vi "Acquire Test.vi"() -> ()   [LabVIEW 2018]
panel:
  out "Waveform Graph":waveform(dbl)(graph)
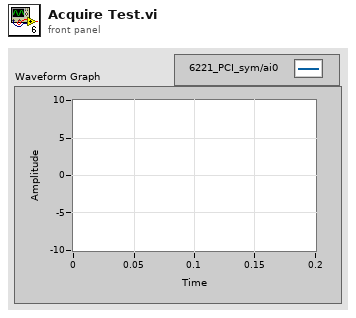
[diagram p1: front panel]
types:
  T1 = typedef "daqtypedef.ctl" = cluster{"PhysicalChanName":tag, "AI.Max":dbl, "AI.Min":dbl, "SampQuant.SampPerChan":dbl, "SampClk.Rate":dbl}
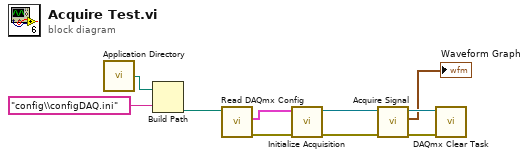
[diagram p0: block diagram]
diagram:
  n1 = call <vilib>:"Application Directory.vi"() -> ("Application Directory"=w10:path)
  n2 = Build Path(base path=w10, name or relative path="config\\configDAQ.ini") -> (appended path=w8:path)
  n3 = call "Read DAQmx Config.vi"("configuration file path"=w8) -> ("error out"=w6:errorcluster, "DAQmx Channel out"=w7:T1)  [unwired: 9 in]
  n4 = call "Initialize Acquisition.vi"("error in"=w6, "DAQmxChannel"=w7) -> ("error out"=w5:errorcluster, "task out"=w4:refnum<k21>)  [unwired: 8 in]
  n5 = call "Acquire Signal.vi"("error in"=w5, "task/channels in"=w4) -> ("error out"=w2:errorcluster, "data"=→"Waveform Graph":waveform(dbl), "task out"=w3:refnum<k21>)  [unwired: 7 in]
  n6 = call <vilib>:"DAQmx Clear Task.vi"("task in"=w3, "error in"=w2) -> ()  [unwired: 13 in, 1 out]
